vi "Update-deposition-status.vi"(8 "error in (no error)":errorcluster, 10 "Status":string, 11 "Data in":T1) -> (0 "error out":errorcluster, 3 "Data out":T1)   [LabVIEW 2013, in "SLMControl.lvlib" / "SC-Main.lvclass"]
uses:
  SC-Main.lvclass
  Object-reference.ctl
  SA-SLMAPI/Sources/Base-statusses.ctl
  UI/Control-names.ctl
  SC-Main.lvclass/SC-Main.ctl
  Enqueue-modes.ctl
  Main-actions.ctl
  Write Deposition status.vi
  Read UI.vi
  UI/Set-control-string.vi
  UI/SC-UI.lvclass
  SA-SLMAPI/SLMAPI.lvlib
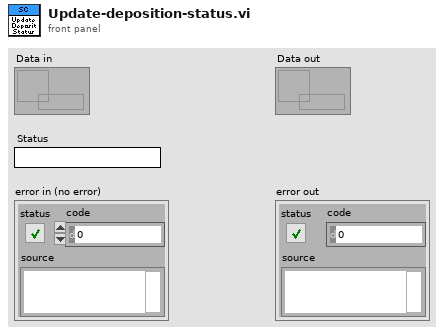
[diagram p1: front panel]
types:
  T1 = typedef "SLMControl.lvlib/SC-Main.lvclass/Object-reference.ctl" = refnum<data-value>
  T2 = typedef "SLMAPI.lvlib/Base-statusses.ctl" = enum16{"Idle", "Initialized", "Configured", "Activated", "Started", "Paused", "Stopped", "Reset", "Error", "Exited"}
  T3 = typedef "SLMControl.lvlib/SC-UI.lvclass/Control-names.ctl" = enum16{"Com-in", "Com-out", "Help", "Status", "Load configuration", "Save configuration", "Load lasing files", "Load deposition files", "Clear", "Files", "Activate", "Execute", "Abort", "Options", "Current layer", "Current iteration", "Last elapsed time", "Deposition status", "Lasing job", "Status LEDs", "Exiting led", "Initialized led", "Files loaded led", "Activated led", "Executing led", "Deposition led", "Lasing job led", "Lasing led"}
  T4 = typedef "SLMControl.lvlib/SC-Main.lvclass/Enqueue-modes.ctl" = enum16{"Default", "Priority", "Flush"}
  T5 = typedef "SLMControl.lvlib/SC-UI.lvclass/Panes-reference.ctl" = refnum<data-value>
  T6 = typedef "SLMControl.lvlib/SC-Main.lvclass/Main-actions.ctl" = enum16{"Idle", "Initialize", "Load configuration", "Save configuration", "Load lasing files", "Load deposition files", "Refresh files", "Clear files", "Open lasing file", "Activate", "Start", "Start deposition cycle", "Start lasing cycle", "Iterate", "Abort", "Stop", "Exit"}
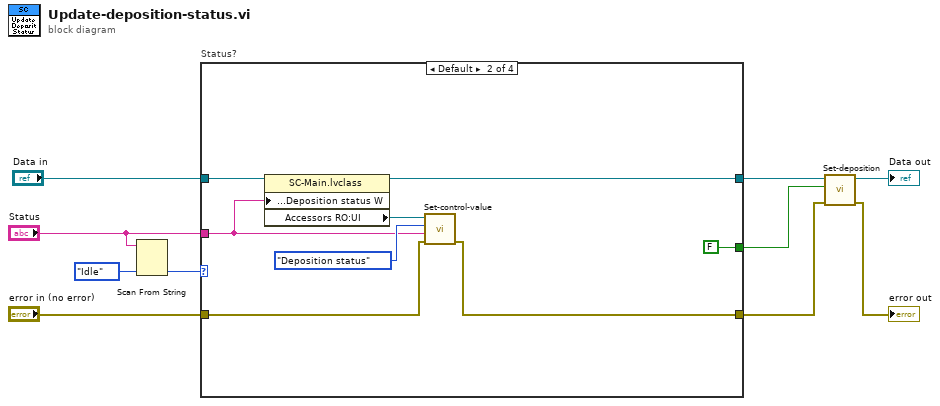
[diagram p0: block diagram]
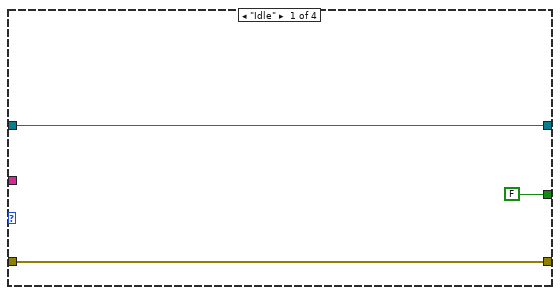
[diagram p2: hidden frame]
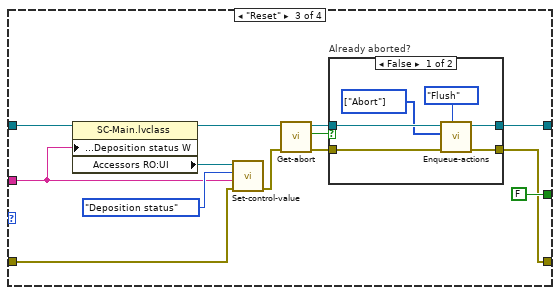
[diagram p3: hidden frame]
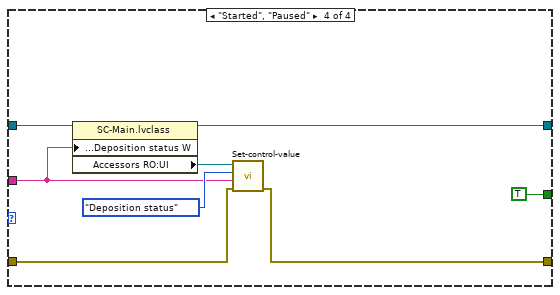
[diagram p5: hidden frame]
diagram:
  n1 = Scan From String(input string="Status", default 1=Base-statusses."Idle" ("Status W")) -> (output 1=w4:T2)  [unwired: 3 in, 3 out]
  n2 = case "Status?" shown="Default" w4 {
    tunnel: "Data in" -> [w13 w21 w34 w50]
    tunnel: [w13 w20 w25 w49] -> w5
    tunnel: "error in (no error)" -> [w11 w14 w28 w43]
    tunnel: [FALSE FALSE FALSE TRUE] -> w8
    tunnel: [w11 w17 w22 w46] -> w9
    tunnel: "Status" -> [_ w15 w29 w44]
    frame "Idle" {
    }
    frame Default {
      n3 = property class="SC-Main.lvclass"(reference=w21, "Accessors/Modifiers:Deposition status W"=w15) -> (reference out=w20:T1, "Accessors RO:UI"=w18:T5)  [unwired: 1 in, 1 out]
      n4 = call-poly "Set-control-value.vi"("error in (no error)"=w14, "Value"=w15, "Control name"=Control-names."Deposition status", "Panes in"=w18) -> ("error out"=w17:errorcluster)  [unwired: 6 in, 1 out]
    }
    frame "Reset" {
      n5 = property class="SC-Main.lvclass"(reference=w34, "Accessors/Modifiers:Deposition status W"=w29) -> (reference out=w33:T1, "Accessors RO:UI"=w31:T5)  [unwired: 1 in, 1 out]
      n6 = call-poly "Set-control-value.vi"("error in (no error)"=w28, "Value"=w29, "Control name"=Control-names."Deposition status", "Panes in"=w31) -> ("error out"=w26:errorcluster)  [unwired: 6 in, 1 out]
      n7 = call "Get-abort.vi"("error in (no error)"=w26, "Object ref in"=w33) -> ("error out"=w23:errorcluster, "Abort"=w24:bool, "Object ref out"=w27:T1)  [unwired: 7 in]
      n8 = case "Already aborted?" shown="False" w24 {
        tunnel: w27 -> [w40 w42]
        tunnel: [w39 w42] -> w25
        tunnel: w23 -> [w37 w41]
        tunnel: [w36 w41] -> w22
        frame False {
          w35 = T6[] [enum."Abort"] items=["Idle", "Initialize", "Load configuration", "Save configuration", "Load lasing files", "Load deposition files", "Refresh files", "Clear files", "Open lasing file", "Activate", "Start", "Start deposition cycle", "Start lasing cycle", "Iterate", "Abort", "Stop", "Exit"] ("State array")
          n9 = call "Enqueue-actions.vi"("Enqueue mode"=Enqueue-modes."Flush", "error in (no error)"=w37, "State array"=w35, "State queue in"=w40) -> ("error out"=w36:errorcluster, "State queue out"=w39:T1)  [unwired: 5 in, 1 out]
        }
        frame True {
        }
      }
    }
    frame "Started", "Paused" {
      n10 = property class="SC-Main.lvclass"(reference=w50, "Accessors/Modifiers:Deposition status W"=w44) -> (reference out=w49:T1, "Accessors RO:UI"=w47:T5)  [unwired: 1 in, 1 out]
      n11 = call-poly "Set-control-value.vi"("error in (no error)"=w43, "Value"=w44, "Control name"=Control-names."Deposition status", "Panes in"=w47) -> ("error out"=w46:errorcluster)  [unwired: 6 in, 1 out]
    }
  }
  n12 = call "Set-deposition.vi"("error in (no error)"=w9, "Depositing?"=w8, "Object ref in"=w5) -> ("error out"=→"error out":errorcluster, "Object ref out"=→"Data out":T1)  [unwired: 7 in]
